vi "Test Create Logger with Queue Sink as Default Config.vi"(11 "Test Case In":refnum<class "Queue Sink.lvclass">) -> (0 "error out":errorcluster, 3 "Test Case Out":refnum<class "Queue Sink.lvclass">)   [LabVIEW 2020, in "Queue Sink.lvclass"]
uses:
  Queue Sink.lvclass
  C:/Program Files (x86)/National Instruments/LabVIEW 2020/vi.lib/Astemes/LUnit/Test Case.lvclass
  Source/Type Defs/Debug Level.ctl
  <vilib>/Astemes/LUnit/Test Case.lvclass/Test Case.ctl
  186b7594-36c3-475d-9f56-112695fdc62a.vi
  9f417576-4e54-4520-bbfc-3f0305dac5bd.vi
  abc007d3-7e1b-4fc8-9ad7-ed682a564c3c.vi
  <vilib>/Astemes/LUnit/Core/LUnit Test Case/Private/Append Pass Result.vi
  <vilib>/Astemes/LUnit/Core/LUnit Test Case/Private/Append Fail Result.vi
  186b7594-36c3-475d-9f56-112695fdc62a.vi/9c5d11cd-9439-4240-a1ee-d9baace9c924.vi
  9f417576-4e54-4520-bbfc-3f0305dac5bd.vi/9c5d11cd-9439-4240-a1ee-d9baace9c924.vi
  abc007d3-7e1b-4fc8-9ad7-ed682a564c3c.vi/9c5d11cd-9439-4240-a1ee-d9baace9c924.vi
  <vilib>/Astemes/LUnit/Core/LUnit Test Case/Private/Run In UI.vi
  <vilib>/Utility/error.llb/Clear Errors.vi
  Source/Sinks/Queue Sink/Queue Sink.lvclass
  C:/Users/hughe_cx/Documents/05_repos/LVLog/Source/Sinks/Sink/Sink.lvclass
  Source/LV Log.lvlib
  Source/Logger/Logger.lvclass
  <vilib>/Astemes/LUnit/Test Case.lvclass
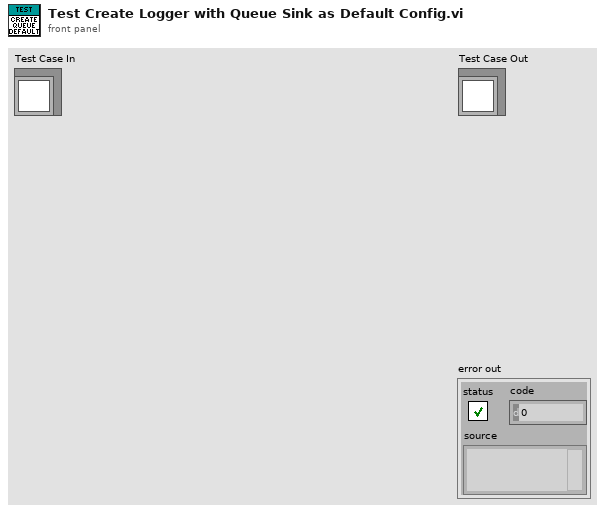
[diagram p1: front panel]
types:
  T1 = typedef "LV Log.lvlib/Debug Level.ctl" = enum16{"DEFAULT", "DEBUG", "INFO", "WARN", "ERROR", "FATAL"}
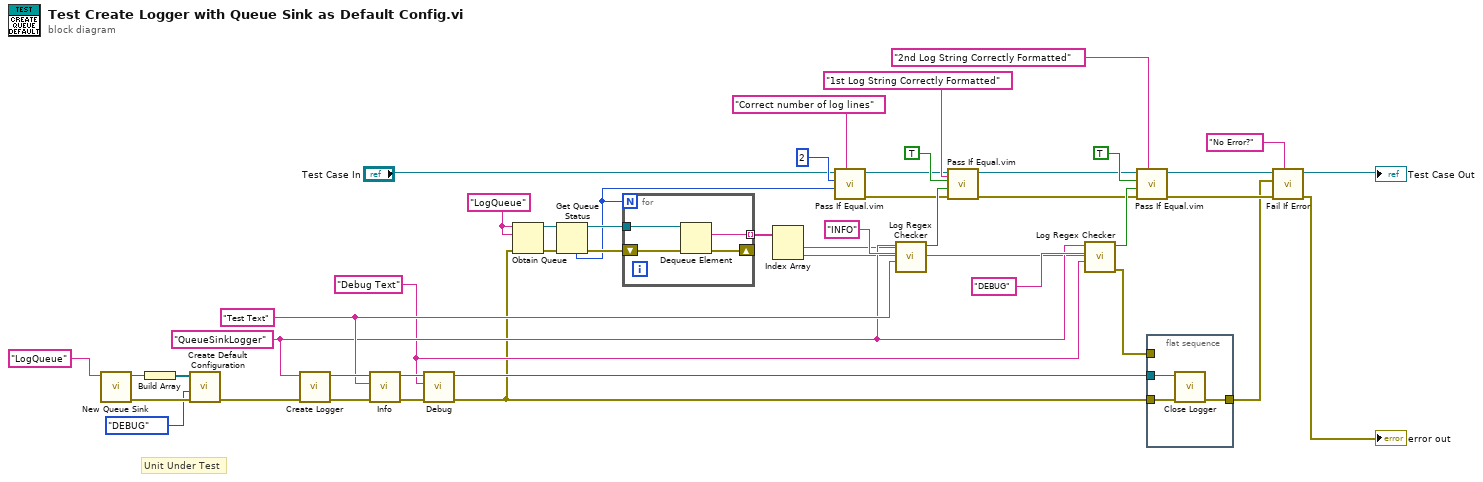
[diagram p0: block diagram]
diagram:
  w13 = "LogQueue" ("name (unnamed)")
  w33 = "Debug Text" ("Log Text")
  w42 = "Test Text" ("Log Text")
  w34 = "QueueSinkLogger" ("Name")
  # "Unit Under Test"
  n1 = call "New Queue Sink.vi"("Queue Name"="LogQueue") -> ("error out"=w4:errorcluster, "Queue Sink out"=w16:refnum<class "Queue Sink.lvclass">)  [unwired: 9 in]
  n2 = Build Array(w16) -> (w2:refnum<class "Queue Sink.lvclass">[])
  n3 = call "Create Default Configuration.vi"("Sinks"=w2, "Debug Level in"=Debug_Level."DEBUG", "error in (no error)"=w4) -> ("error out"=w3:errorcluster)  [unwired: 7 in]
  n4 = call "Create Logger.vi"("error in (no error)"=w3, "Name"=w34) -> ("error out"=w46:errorcluster, "Logger out"=w45:refnum<class "Logger.lvclass">)  [unwired: 8 in]
  n5 = call "Info.vi"("error in (no error)"=w46, "Log Text"=w42, "Logger in"=w45) -> ("error out"=w41:errorcluster, "Logger out"=w40:refnum<class "Logger.lvclass">)  [unwired: 6 in, 1 out]
  n6 = call "Debug.vi"("error in (no error)"=w41, "Log Text"=w33, "Logger in"=w40) -> ("error out"=w5:errorcluster, "Logger out"=w23:refnum<class "Logger.lvclass">)  [unwired: 6 in, 1 out]
  n7 = Obtain Queue(name (unnamed)=w13, element data type=w13, error in (no error)=w5) -> (queue out=w9:refnum<queue>, error out=w10:errorcluster)  [unwired: 2 in, 1 out]
  n8 = Get Queue Status(queue=w9, error in (no error)=w10) -> (queue out=w12:refnum<queue>, error out=w11:errorcluster, # elements in queue=w8:i32)  [unwired: 1 in, 5 out]
  n9 = for {
    N: w8 -> [_]
    shift-right: [w48] -> _
    shift-left: w11 -> [w50]
    tunnel: w12 -> [w49]
    tunnel: [w47] -> w7 mode=indexing
    n10 = Dequeue Element(queue=w49, error in (no error)=w50) -> (element=w47:string, error out=w48:errorcluster)  [unwired: 1 in, 2 out]
  }
  n11 = Index Array(array=w7) -> (element #1=w32:string, element #2=w31:string)  [unwired: 2 in]
  n12 = call "Pass If Equal.vim"("Description"="Correct number of log lines", "Actual"=w8, "Expected"=2, "LUnit Test Case In"="Test Case In") -> ("error out"=w24:errorcluster, "LUnit Test Case Out"=w28:refnum<class "Queue Sink.lvclass">)  [unwired: 6 in]
  n13 = call "Log Regex Checker.vi"("Log String"=w32, "Expected Log Text (Any)"=w42, "Expected Log Level (Any)"="INFO", "Expected Logger Name (Any)"=w34) -> ("Math Found"=w38:bool)  [unwired: 5 in, 2 out]
  n14 = call "Pass If Equal.vim"("Description"="1st Log String Correctly Formatted", "error in (no error)"=w24, "Actual"=w38, "Expected"=TRUE, "LUnit Test Case In"=w28) -> ("error out"=w25:errorcluster, "LUnit Test Case Out"=w30:refnum<class "Queue Sink.lvclass">)  [unwired: 5 in]
  n15 = call "Log Regex Checker.vi"("Log String"=w31, "Expected Log Text (Any)"=w33, "Expected Log Level (Any)"="DEBUG", "Expected Logger Name (Any)"=w34) -> ("error out"=w6:errorcluster, "Math Found"=w37:bool)  [unwired: 5 in, 1 out]
  n16 = call "Pass If Equal.vim"("Description"="2nd Log String Correctly Formatted", "error in (no error)"=w25, "Actual"=w37, "Expected"=TRUE, "LUnit Test Case In"=w30) -> ("error out"=w26:errorcluster, "LUnit Test Case Out"=w29:refnum<class "Queue Sink.lvclass">)  [unwired: 5 in]
  n17 = flat-sequence {
    tunnel: w5 -> [w53]
    tunnel: w23 -> [w52]
    tunnel: [w51] -> w22
    tunnel: w6 -> [_]
    frame #0 {
      n18 = call "Close Logger.vi"("error in (no error)"=w53, "Logger in"=w52) -> ("error out"=w51:errorcluster)  [unwired: 9 in]
    }
  }
  n19 = call <vilib>:"Fail If Error.vi"("Description"="No Error?", "error in (no error)"=w26, "Assert error"=w22, "LUnit Test Case In"=w29) -> ("error out"=→"error out":errorcluster, "LUnit Test Case Out"=→"Test Case Out":refnum<class "Queue Sink.lvclass">)  [unwired: 6 in]
